vi "Create_Destinations.vi"(8 "error in (no error)":errorcluster, 11 "Build in":refnum<class "AB_Application.lvclass">) -> (0 "error out":errorcluster, 2 "createdDirectories":path[](array[path]), 3 "Build out":refnum<class "AB_Application.lvclass">)   [LabVIEW 2020, in "AB_Application.lvclass"]
uses:
  <vilib>/AppBuilder/AB_Classes/Application/AB_Application.lvclass
  e:/builds/penguin/labview/branches/2020/dev/dist/vi.lib/AppBuilder/AB_Classes/TargetFile/AB_Targetfile.lvclass
  <resource>/Framework/Providers/Common/provcom_StringGlobals.vi
  <vilib>/AppBuilder/AB_Classes/TargetFile/AB_Targetfile.lvclass
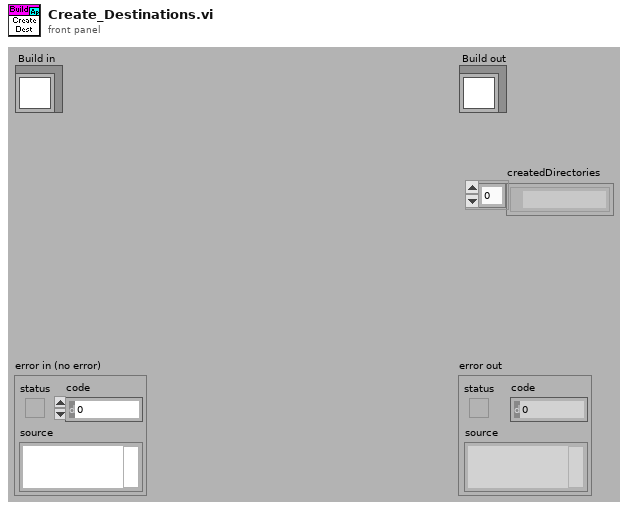
[diagram p1: front panel]
types:
  T1 = typedef "AB_Targetfile.ctl" = cluster{"targetfileName":string, "targetfileGUID":string, "enableDebugging":bool, "versionInfo":cluster{"productName":string, "legalCopyright":string, "companyName":string, "internalName":string, "fileDescription":string}, "eng_consolidatedTypeInfo":string, "fastFileFormat":bool, "eng_LEIFBuildData":u32, "versionIndependent":bool}
  T2 = enum32{"invalid OS target", "Mac OS", "Windows 3.1", "Windows 95/NT", "Solaris 1", "Solaris 2", "HP-UX", "PowerMAX", "Linux", "Irix", "Rhapsody", "BeOS", "AIX", "OSF1", "VxWorks", "PharLap", "Carbon", "RTX", "Windows x64", "Linux x64", "Mac OS X x64"}
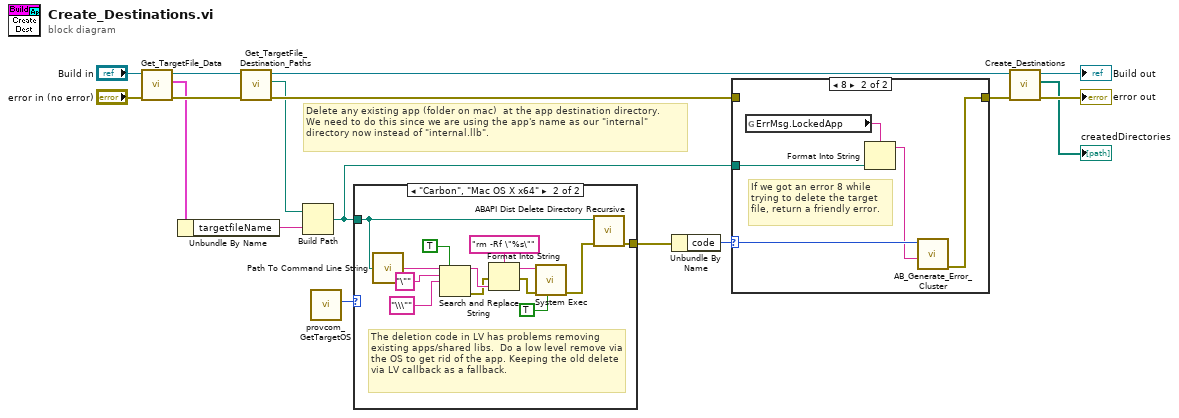
[diagram p0: block diagram]
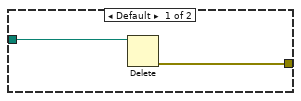
[diagram p3: hidden frame]
diagram:
  # "Delete any existing app (folder on mac)  at the app destination directory.\nWe need to do this since we are using the app's name as our \"internal\" directory now instead of \"internal.llb\"."
  n1 = call <vilib>:"Get_TargetFile_Data.vi"("error in (no error)"="error in (no error)", "AB_Targetfile in"="Build in") -> ("error out"=w10:errorcluster, "data"=w8:T1, "AB_Targetfile out"=w9:refnum<class "AB_Application.lvclass">)  [unwired: 7 in]
  n2 = Unbundle By Name(w8) -> ("targetfileName"=w13:string)
  n3 = call <vilib>:"Get_TargetFile_Destination_Paths.vi"("error in (no error)"=w10, "AB_Targetfile in"=w9) -> ("error out"=w6:errorcluster, "destination path"=w4:path, "AB_Targetfile out"=w14:refnum<class "AB_Application.lvclass">)  [unwired: 5 in, 2 out]
  n4 = Build Path(base path=w4, name or relative path=w13) -> (appended path=w3:path)
  n5 = call <resource>:"provcom_GetTargetOS.vi"() -> ("App.TargetOS"=w7:T2)  [unwired: 11 out]
  n6 = case shown="\"Carbon\", \"Mac OS X x64\"" w7 {
    tunnel: w3 -> [w19 w31]
    tunnel: [w18 w32] -> w2
    frame Default {
      n7 = Delete(path (use dialog)=w19) -> (error out=w18:errorcluster)  [unwired: 1 in, 5 out]
    }
    frame "Carbon", "Mac OS X x64" {
      # "The deletion code in LV has problems removing existing apps/shared libs.  Do a low level remove via the OS to get rid of the app. Keeping the old delete via LV callback as a fallback."
      n8 = call <vilib>:"Path To Command Line String.vi"("path"=w31) -> ("string"=w25:string)
      n9 = Search and Replace String(replace all?=TRUE ("replace all? (F)"), input string=w25, search string="\"" ("replace string (\"\")"), replace string="\\\"" ("replace string (\"\")")) -> (result string=w23:string, error out=w21:errorcluster)  [unwired: 4 in, 2 out]
      n10 = Format Into String(format string="rm -Rf \"%s\"", error in=w21, w23) -> (resulting string=w22:string, error out=w20:errorcluster)  [unwired: 1 in]
      n11 = call <vilib>:"System Exec.vi"("run minimized? (F)"=TRUE, "error in (no error)"=w20, "command line"=w22) -> ("error out"=w26:errorcluster)  [unwired: 5 in, 3 out]
      n12 = call <vilib>:"ABAPI Dist Delete Directory Recursive.vi"("error in (no error)"=w26, "directory"=w31) -> ("error out"=w32:errorcluster)  [unwired: 9 out]
    }
  }
  n13 = Unbundle By Name(w2) -> ("code"=w1:i32)
  n14 = case shown="8" w1 {
    selector: w1 -> [_ w38]
    tunnel: w6 -> [w33 _]
    tunnel: [w33 w37] -> w5
    tunnel: w3 -> [_ w34]
    frame Default {
      # "Since we're always deleting, don't return any other errors (such as error 7)."
    }
    frame 8 {
      # "If we got an error 8 while trying to delete the target file, return a friendly error."
      n15 = global read "provcom_StringGlobals.vi" "ErrMsg.LockedApp"() -> (w36:string)
      n16 = Format Into String(format string=w36, w34) -> (resulting string=w35:string)  [unwired: 2 in, 1 out]
      n17 = call <vilib>:"AB_Generate_Error_Cluster.vi"("Additional Message"=w35, "Code"=w38) -> ("error out"=w37:errorcluster)  [unwired: 2 in, 7 out]
    }
  }
  n18 = call-parent "Create_Destinations.vi"("error in (no error)"=w5, "Build in"=w14) -> ("error out"=→"error out":errorcluster, "createdDirectories"=→"createdDirectories":path[], "Build out"=→"Build out":refnum<class "AB_Application.lvclass">)  [unwired: 7 out]
